vi "Query Sys (To) Parameters (Input).vi"(8 "error in (no error)":errorcluster, 11 "VISA resource name":refnum<visa-resource-name>) -> (0 "error out":errorcluster, 2 "Input Parameters":T1={"Sys Ext Mode"=enum."Disabled", "Trig Level"=2.5, "Trig Edge"=TRUE, "Gate Logic"=TRUE, "Gate Level"=2.5, "Gate Mode"=enum."Disabled"} {"Gate Level" format="%.4p"; "Trig Level" format="%.4p"}, 3 "VISA resource name out":refnum<visa-resource-name>)   [LabVIEW 2012, in "Quantum Composers 9000 Series.lvlib"]
doc: "This VI is used to read the input configuration of the system timer (To)."
uses:
  Quantum Composers 9000 Series.lvlib
panel:
  # "Triggered"
  # "Gated"
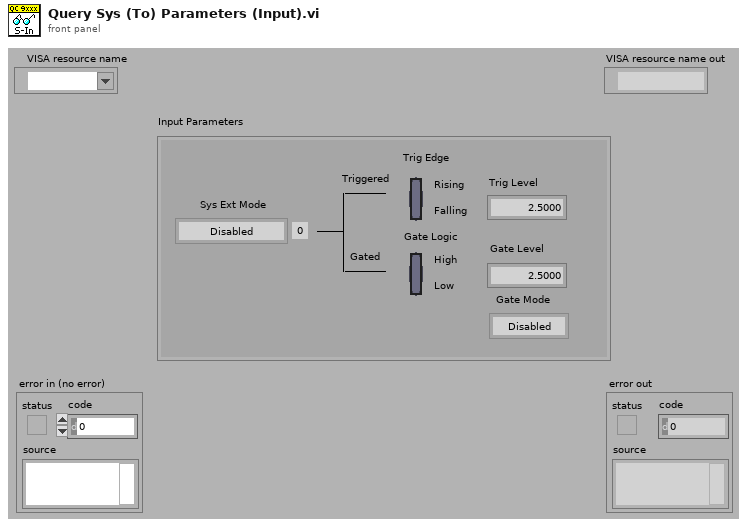
[diagram p1: front panel]
types:
  T1 = cluster{"Sys Ext Mode":enum16{"Disabled", "Triggered", "Gated", "Triggered & Gated"}, "Trig Level":dbl, "Trig Edge":bool, "Gate Logic":bool, "Gate Level":dbl, "Gate Mode":enum16{"Disabled", "Pulse Inhibit", "Output Inhibit", "Channel"}}
  T2 = enum16{"Disabled", "Triggered", "Gated", "Triggered & Gated"}
  T3 = enum16{"Disabled", "Pulse Inhibit", "Output Inhibit", "Channel"}
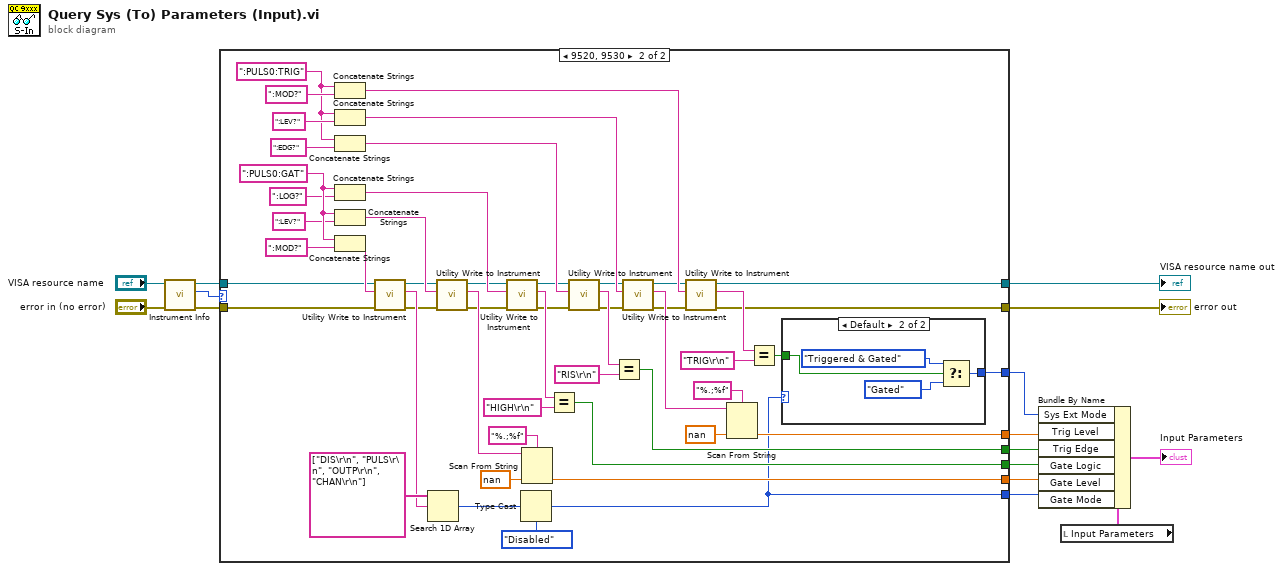
[diagram p0: block diagram]
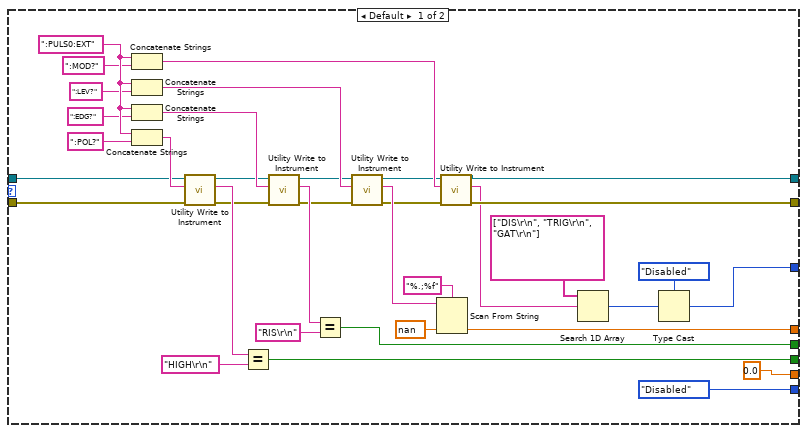
[diagram p2: hidden frame]
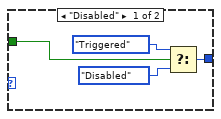
[diagram p3: hidden frame]
diagram:
  n1 = call "Instrument Info.vi"("error in (no error)"="error in (no error)", "VISA resource name"="VISA resource name") -> ("error out"=w8:errorcluster, "Instr Model"=w1:u32, "VISA resource name out"=w9:refnum<visa-resource-name>)  [unwired: 7 out]
  n2 = case shown="9520, 9530" w1 {
    tunnel: [w51 w60] -> w15
    tunnel: [w50 w59] -> w14
    tunnel: [w48 w101] -> w6
    tunnel: [w18 w52] -> w2
    tunnel: [w41 w98] -> w5
    tunnel: [w38 w96] -> w7
    tunnel: w9 -> [w22 w69]
    tunnel: w8 -> [w21 w70]
    tunnel: [T3."Disabled" ("Gate Mode") w54] -> w3
    tunnel: [0.0 ("Gate Level") w79] -> w4
    frame Default {
      w33 = ":PULS0:EXT"
      n3 = Concatenate Strings(w33, ":MOD?") -> (w47:string)
      n4 = Concatenate Strings(w33, ":LEV?") -> (w36:string)
      n5 = Concatenate Strings(w33, ":EDG?") -> (w37:string)
      n6 = Concatenate Strings(w33, ":POL?") -> (w44:string)
      n7 = call "Utility Write to Instrument.vi"("error in (no error)"=w21, "Write Buffer"=w44, "VISA resource name"=w22) -> ("error out"=w24:errorcluster, "Read Buffer"=w43:string, "VISA resource name out"=w23:refnum<visa-resource-name>)  [unwired: 6 out]
      n8 = Equal?(x=w43, y="HIGH\r\n") -> (x = y?=w41:bool)
      n9 = call "Utility Write to Instrument.vi"("error in (no error)"=w24, "Write Buffer"=w37, "VISA resource name"=w23) -> ("error out"=w25:errorcluster, "Read Buffer"=w39:string, "VISA resource name out"=w26:refnum<visa-resource-name>)  [unwired: 6 out]
      n10 = Equal?(x=w39, y="RIS\r\n") -> (x = y?=w38:bool)
      n11 = call "Utility Write to Instrument.vi"("error in (no error)"=w25, "Write Buffer"=w36, "VISA resource name"=w26) -> ("error out"=w28:errorcluster, "Read Buffer"=w35:string, "VISA resource name out"=w27:refnum<visa-resource-name>)  [unwired: 6 out]
      n12 = Scan From String(format string="%.;%f", input string=w35, default 1=nan ("default value 1")) -> (output 1=w48:dbl)  [unwired: 2 in, 3 out]
      n13 = call "Utility Write to Instrument.vi"("error in (no error)"=w28, "Write Buffer"=w47, "VISA resource name"=w27) -> ("error out"=w50:errorcluster, "Read Buffer"=w45:string, "VISA resource name out"=w51:refnum<visa-resource-name>)  [unwired: 6 out]
      n14 = Search 1D Array(1D array=string[] ["DIS\r\n", "TRIG\r\n", "GAT\r\n"], element=w45) -> (index of element=w17:i32)  [unwired: 1 out]
      n15 = Type Cast(type=T2."Disabled" ("Sys Ext Mode"), x=w17) -> (*(type *) &x=w18:T2)
    }
    frame 9520, 9530 {
      w85 = ":PULS0:TRIG"
      w92 = ":PULS0:GAT"
      n16 = Concatenate Strings(w85, ":MOD?") -> (w84:string)
      n17 = Concatenate Strings(w85, ":LEV?") -> (w82:string)
      n18 = Concatenate Strings(w85, ":EDG?") -> (w83:string)
      n19 = Concatenate Strings(w92, ":LOG?") -> (w94:string)
      n20 = Concatenate Strings(w92, ":LEV?") -> (w95:string)
      n21 = Concatenate Strings(w92, ":MOD?") -> (w100:string)
      n22 = call "Utility Write to Instrument.vi"("error in (no error)"=w70, "Write Buffer"=w100, "VISA resource name"=w69) -> ("error out"=w68:errorcluster, "Read Buffer"=w71:string, "VISA resource name out"=w67:refnum<visa-resource-name>)  [unwired: 6 out]
      n23 = Search 1D Array(1D array=string[] ["DIS\r\n", "PULS\r\n", "OUTP\r\n", "CHAN\r\n"], element=w71) -> (index of element=w56:i32)  [unwired: 1 out]
      n24 = call "Utility Write to Instrument.vi"("error in (no error)"=w68, "Write Buffer"=w95, "VISA resource name"=w67) -> ("error out"=w66:errorcluster, "Read Buffer"=w78:string, "VISA resource name out"=w65:refnum<visa-resource-name>)  [unwired: 6 out]
      n25 = call "Utility Write to Instrument.vi"("error in (no error)"=w66, "Write Buffer"=w94, "VISA resource name"=w65) -> ("error out"=w64:errorcluster, "Read Buffer"=w76:string, "VISA resource name out"=w63:refnum<visa-resource-name>)  [unwired: 6 out]
      n26 = Type Cast(type=T3."Disabled" ("Gate Mode"), x=w56) -> (*(type *) &x=w54:T3)
      n27 = Scan From String(format string="%.;%f", input string=w78, default 1=nan ("default value 1")) -> (output 1=w79:dbl)  [unwired: 2 in, 3 out]
      n28 = Equal?(x=w76, y="HIGH\r\n") -> (x = y?=w98:bool)
      n29 = call "Utility Write to Instrument.vi"("error in (no error)"=w64, "Write Buffer"=w83, "VISA resource name"=w63) -> ("error out"=w57:errorcluster, "Read Buffer"=w75:string, "VISA resource name out"=w62:refnum<visa-resource-name>)  [unwired: 6 out]
      n30 = Equal?(x=w75, y="RIS\r\n") -> (x = y?=w96:bool)
      n31 = call "Utility Write to Instrument.vi"("error in (no error)"=w57, "Write Buffer"=w82, "VISA resource name"=w62) -> ("error out"=w58:errorcluster, "Read Buffer"=w77:string, "VISA resource name out"=w61:refnum<visa-resource-name>)  [unwired: 6 out]
      n32 = call "Utility Write to Instrument.vi"("error in (no error)"=w58, "Write Buffer"=w84, "VISA resource name"=w61) -> ("error out"=w59:errorcluster, "Read Buffer"=w73:string, "VISA resource name out"=w60:refnum<visa-resource-name>)  [unwired: 6 out]
      n33 = Scan From String(format string="%.;%f", input string=w77, default 1=nan ("default value 1")) -> (output 1=w101:dbl)  [unwired: 2 in, 3 out]
      n34 = Equal?(x=w73, y="TRIG\r\n") -> (x = y?=w53:bool)
      n35 = case shown="Default" w54 {
        tunnel: w53 -> [w104 w108]
        tunnel: [w103 w107] -> w52
        frame "Disabled" {
          n36 = Select(t=T2."Triggered" ("Sys Ext Mode"), s=w104, f=T2."Disabled" ("Sys Ext Mode")) -> (s? t:f=w103:T2)
        }
        frame Default {
          n37 = Select(t=T2."Triggered & Gated" ("Sys Ext Mode"), s=w108, f=T2."Gated" ("Sys Ext Mode")) -> (s? t:f=w107:T2)
        }
      }
    }
  }
  "VISA resource name out" <- w15
  "error out" <- w14
  n38 = local read "Input Parameters"() -> (w12:T1)
  n39 = Bundle By Name(cluster=w12, "Sys Ext Mode"=w2, "Trig Level"=w6, "Trig Edge"=w7, "Gate Logic"=w5, "Gate Level"=w4, "Gate Mode"=w3) -> (→"Input Parameters":T1)
